vi "XiXi-1(Add DBL，利用索引数组).vi"(10 "X[-1]":dbl, 11 "Xi":dbl[](array[numeric])) -> (3 "Yi":dbl[](array[numeric]) format="%.2f")   [LabVIEW 2012]
doc: "Calculate sums of consecutive array elements. 0th element of output is equal to x(0)+ x(-1), where x(-1) is an optional scalar input that defaults to zero."
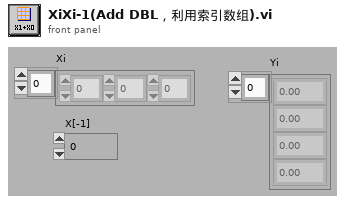
[diagram p1: front panel]
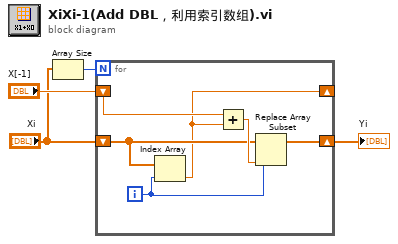
[diagram p0: block diagram]
diagram:
  n1 = Array Size(array="Xi") -> (size(s)=w1:i32)
  n2 = for {
    N: w1 -> [_]
    shift-right: [w10] -> w3
    shift-left: "Xi" -> [w7]
    shift-right: [w5] -> _
    shift-left: "X[-1]" -> [w9]
    i -> [w6]
    n3 = Index Array(array=w7, index=w6) -> (element=w5:dbl)
    n4 = Add(x=w9, y=w5) -> (x+y=w8:dbl)
    n5 = Replace Array Subset(array=w7, new element=w8, index=w6) -> (w10:dbl[])
  }
  "Yi" <- w3
